vi "Unpack Message.vi"(8 "error in (no error)":errorcluster, 9 "Packed Message":string, 10 "Message Name":string, 11 "Car Wash Option Finished in":refnum<class "Car Wash Option Finished.lvclass">) -> (0 "error out":errorcluster, 2 "Valid":bool, 3 "Car Wash Option Finished out":refnum<class "Car Wash Option Finished.lvclass">)   [LabVIEW 2016, in "CLD Exam - Car Wash.lvlib" / "Car Wash Option Finished.lvclass"]
uses:
  Car Wash Option Finished.lvclass
  Mediator/Classes/Message Data Interface/Data Message Interface.lvclass
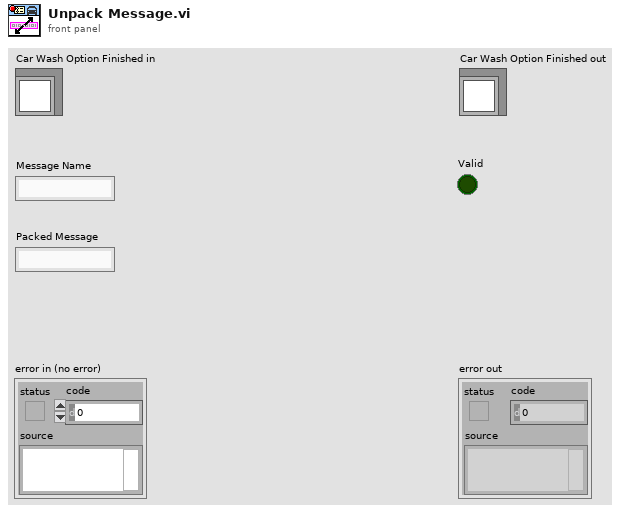
[diagram p1: front panel]
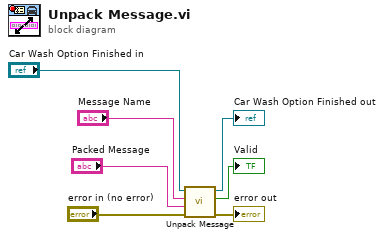
[diagram p0: block diagram]
diagram:
  n1 = call-parent "Unpack Message.vi"("error in (no error)"="error in (no error)", "Packed Message"="Packed Message", "Message Name"="Message Name", "Data Message Interface in"="Car Wash Option Finished in") -> ("error out"=→"error out":errorcluster, "Valid"=→"Valid":bool, "Data Message Interface out"=→"Car Wash Option Finished out":refnum<class "Car Wash Option Finished.lvclass">)  [unwired: 5 in]
